vi "Periodic Tasks.vi"(8 "error in":errorcluster) -> ()   [LabVIEW 2019]
doc: "This VI runs in parallel to other tasks. It can contain as many user-defined periodic loops as you need. These can carry out PID or other sorts of timed response."
uses:
  <vilib>/Rock Robotics/WPI/ThirdParty/Phoenix-LabVIEW/Motor Controller/Controls/CTRE_Phoenix_MotorControl_ControlMode.ctl
  <vilib>/Rock Robotics/WPI/Utilities/WPI_GetSetVariantRefNum.vi
  <vilib>/Rock Robotics/Network Tables/NT Read Number.vi
  <vilib>/Rock Robotics/WPI/ThirdParty/Phoenix-LabVIEW/Motor Controller/Get/CTRE_Phoenix_MotorController_GetSupplyAndStatorCurrent_Enhanced.vi
  <vilib>/Rock Robotics/WPI/ThirdParty/Phoenix-LabVIEW/Motor Controller/Get/CTRE_Phoenix_MotorController_GetSelectedSensorData.vi
  <vilib>/gmath/NI_Gmath.lvlib
panel:
  in  "Output":dbl
  out "Target RPM":dbl
  out "Rpm":cluster{dbl, "Target RPM":dbl}(graph)
  out "Current":T1(graph)
  in  "PIDF Slot":i32
  in  "I-Zone":dbl
  in  "F":dbl=0.055
  in  "D":dbl
  in  "I":dbl
  in  "P":dbl
  out "Target Dist":dbl
  out "Outtake Sensor":bool
  out "Intake Sensor":bool
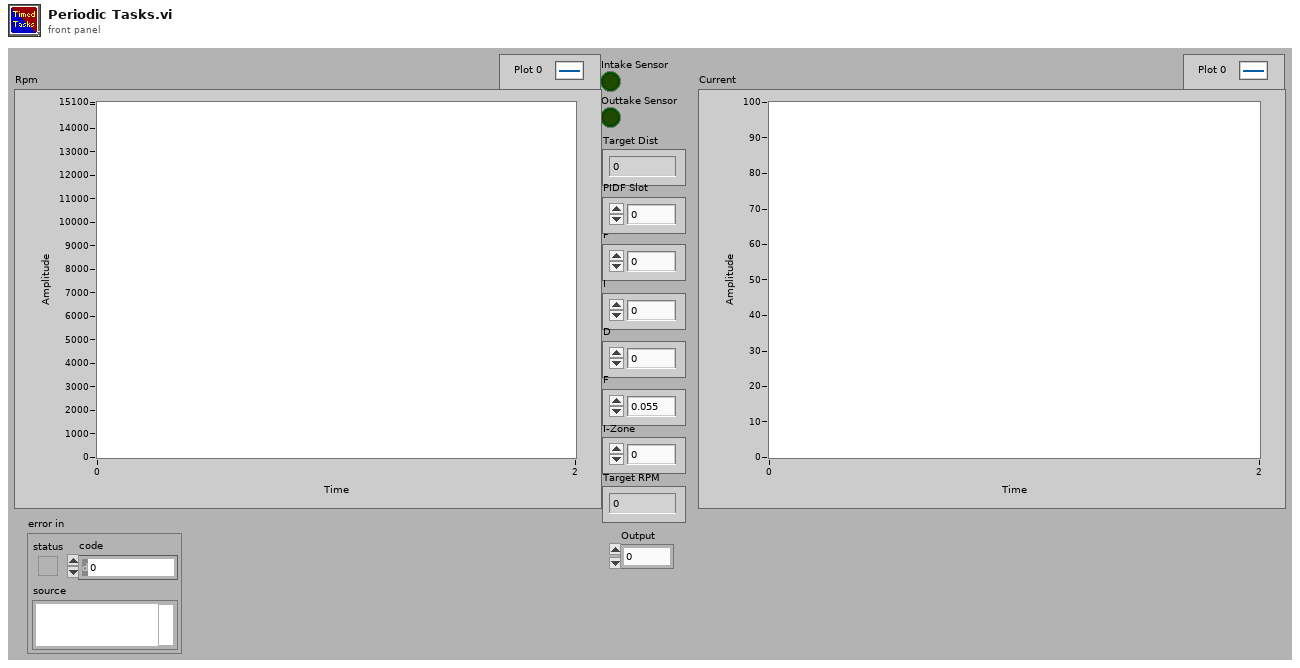
[diagram p1: front panel]
types:
  T1 = cluster{"Supply Current":dbl, "Stator Current":dbl}
  T2 = typedef "WPI_JoystickDevRef.ctl" = cluster{"Device":T3}
  T3 = typedef "WPI_JoystickDeviceEnum.ctl" = enum16{"USB 0", "USB 1", "USB 2", "USB 3", "USB 4", "USB 5"}
  T4 = typedef "WPI_MotorControlDeviceRef.ctl" = cluster{"DeviceStatus":errorcluster, "Type":T5, "PWM":cluster{"PWM Channel":T6, "DeadBand":T7}, "CAN":cluster{"Device Number":u8, "SetOutput VI Ref":variant, "GetOutput VI Ref":variant, "Enable VI Ref":variant, "Disable VI Ref":variant, "Data":variant}, "Invert":bool, "DIO PWM":cluster{"PWM \"Enable\" Channel":T6, "DIOChannel":T8, "PWM Rate":dbl}}
  T5 = typedef "WPI_MotorControlType.ctl" = enum16{"PWM", "CAN", "DIO PWM"}
  T6 = typedef "FPGA_DIOPWMChannel.ctl" = enum8{"PWM 0", "PWM 1", "PWM 2", "PWM 3", "PWM 4", "PWM 5", "PWM 6", "PWM 7", "PWM 8", "PWM 9", "PWM MXP 0", "PWM MXP 1", "PWM MXP 2", "PWM MXP 3", "PWM MXP 4", "PWM MXP 5", "PWM MXP 6", "PWM MXP 7", "PWM MXP 8", "PWM MXP 9", "Invalid"}
  T7 = typedef "WPI_PWMDeadband.ctl" = cluster{"Name":string, "maxPositivePwm":i32, "minPositivePwm":i32, "centerPwm":i32, "maxNegativePwm":i32, "minNegativePwm":i32, "angularRange":u16}
  T8 = typedef "FPGA_DIOChannel.ctl" = enum8{"DIO 0", "DIO 1", "DIO 2", "DIO 3", "DIO 4", "DIO 5", "DIO 6", "DIO 7", "DIO 8", "DIO 9", "DIO MXP 0", "DIO MXP 1", "DIO MXP 2", "DIO MXP 3", "DIO MXP 4", "DIO MXP 5", "DIO MXP 6", "DIO MXP 7", "DIO MXP 8", "DIO MXP 9", "DIO MXP 10", "DIO MXP 11", "DIO MXP 12", "DIO MXP 13", "DIO MXP 14", "DIO MXP 15", "SPI Port CS1", "SPI Port CS2", "SPI Port CS3", "SPI Port MISO", "SPI Port MOSI", "Invalid"}
  T9 = cluster{"PhoenixMotorControlDevRef":T4, "JoystickDevRef":T2}
  T10 = typedef "CTRE_Phoenix_MotorControl_ControlMode.ctl" = u16
  T11 = typedef "WPI_DigitalInputDevRef.ctl" = cluster{"DevStatus":errorcluster, "DIO Channel":T8}
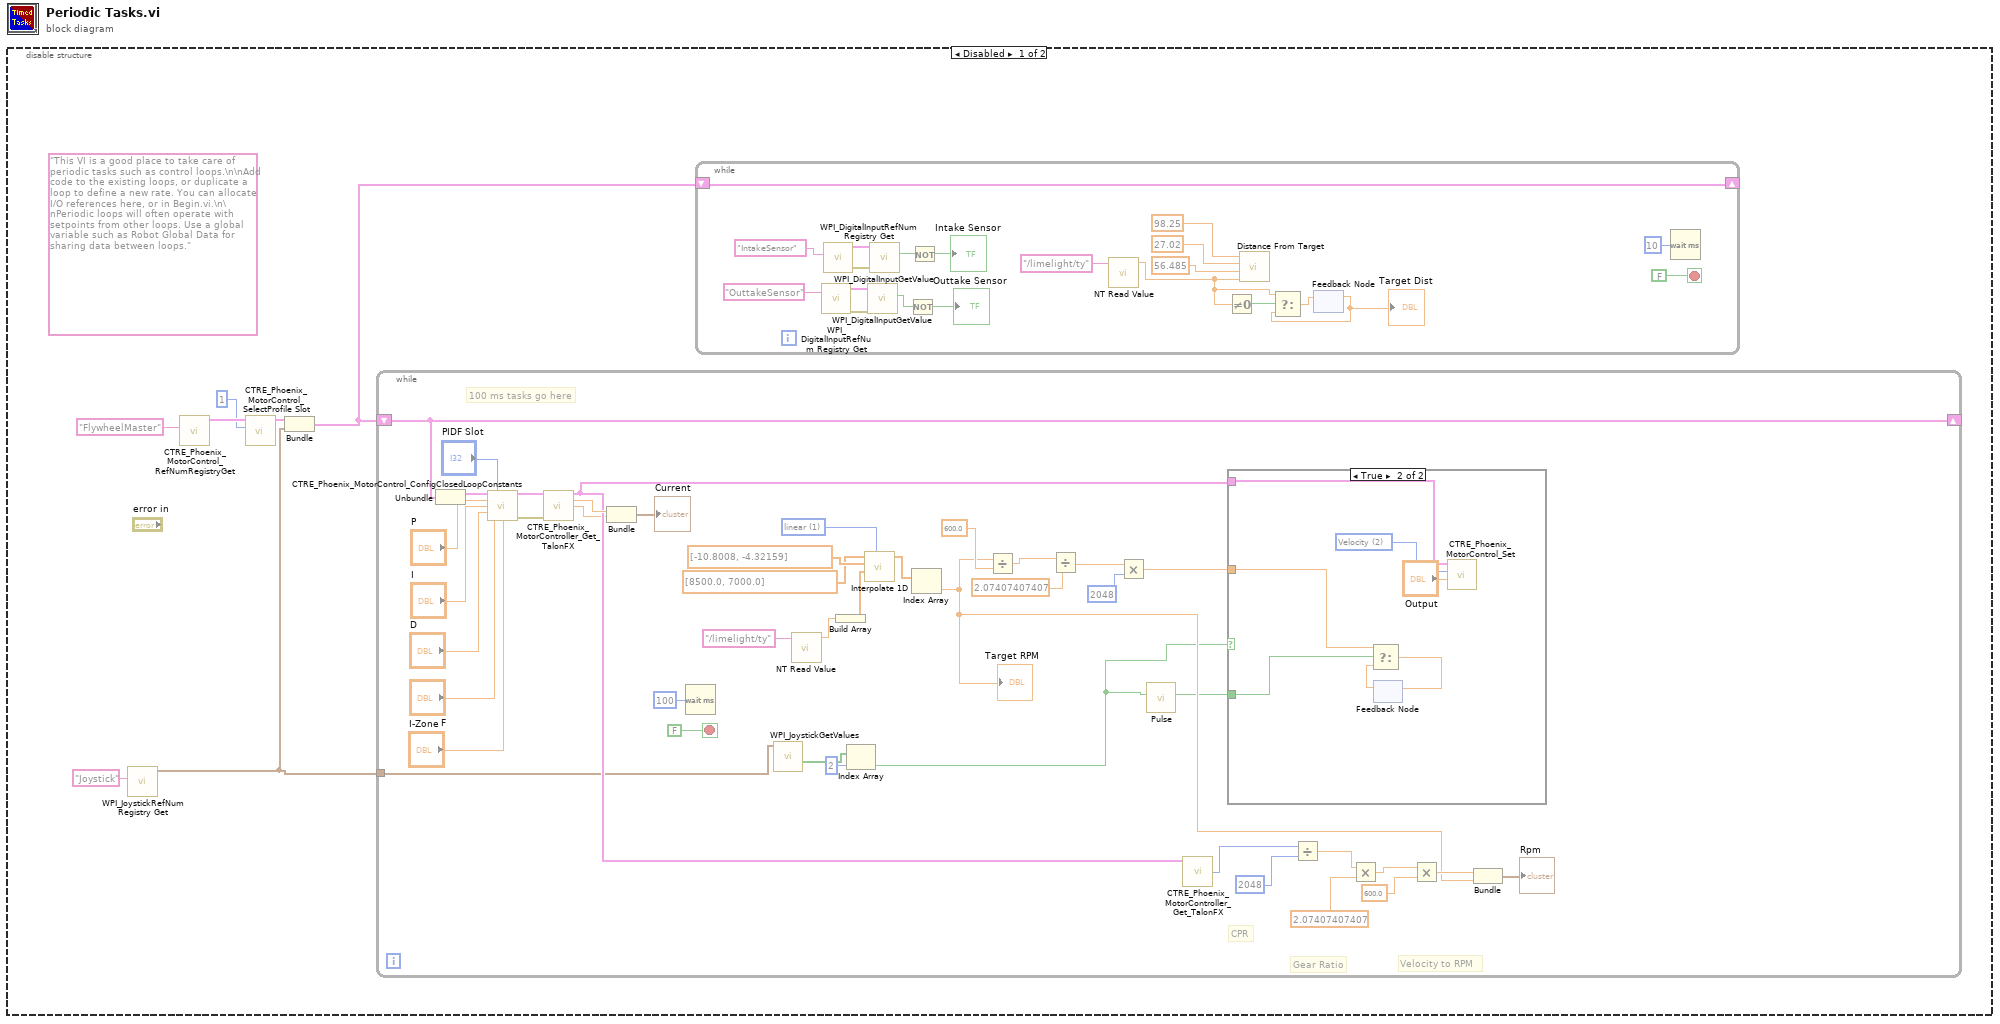
[diagram p0: block diagram]
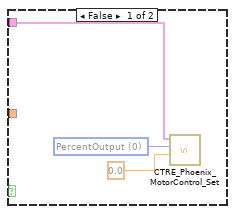
[diagram p2: hidden frame]
diagram:
  n1 = disable-structure shown="Disabled" {
    frame Disabled {
      (unwired) "This VI is a good place to take care of periodic tasks such as control loops.\n\nAdd code to the existing loops, or duplicate a loop to define a new rate. You can allocate I/O references here, or in Begin.vi.\n\nPeriodic loops will often operate with setpoints from other loops. Use a global variable such as Robot Global Data for sharing data between loops."
      n2 = call <vilib>:"WPI_JoystickRefNum Registry Get.vi"("refnum name"="Joystick") -> ("JoystickDevRef"=w1:T2)  [unwired: 9 in, 1 out]
      n3 = call <vilib>:"CTRE_Phoenix_MotorControl_RefNumRegistryGet.vi"("refnum name"="FlywheelMaster") -> ("PhoenixMotorControlDevRef"=w5:T4)  [unwired: 9 in, 1 out]
      n4 = call <vilib>:"CTRE_Phoenix_MotorControl_SelectProfile Slot.vi"("slotIdx"=1, "PhoenixMotorControlDevRef"=w5) -> ("PhoenixMotorControlDevRef"=w4:T4)  [unwired: 8 in, 1 out]
      n5 = Bundle("PhoenixMotorControlDevRef"=w4, "JoystickDevRef"=w1) -> (w7:T9)  [unwired: 1 out]
      n6 = while {
        shift-right: [w48] -> _
        shift-left: w7 -> [w48]
        tunnel: w1 -> [w13]
        stop <- FALSE stop-if-true
        w21 = 1 items=["nearest", "linear", "spline", "cubic Hermite", "Lagrange"] ("method")
        # "CPR"
        # "Velocity to RPM"
        # "Gear Ratio"
        # "100 ms tasks go here"
        n7 = Unbundle(w48) -> ("PhoenixMotorControlDevRef"=w47:T4)  [unwired: 1 out]
        n8 = call <vilib>:"CTRE_Phoenix_MotorControl_ConfigClosedLoopConstants.vi"("PhoenixMotorControlDevRef"=w47, "slotIdx"="PIDF Slot", "P"="P", "I"="I", "D"="D", "F"="F", "I Zone"="I-Zone") -> ("PhoenixMotorControlDevRef"=w40:T4, "error out"=w39:errorcluster)  [unwired: 7 in]
        n9 = call-poly <vilib>:"CTRE_Phoenix_MotorController_Get_TalonFX.vi"("PhoenixMotorControlDevRef"=w40, "error in"=w39) -> ("PhoenixMotorControlDevRef"=w36:T4, "Supply Current"=w37:dbl, "Stator Current"=w35:dbl)  [unwired: 10 in, 1 out]
        n10 = Bundle("Supply Current"=w37, "Stator Current"=w35) -> (→"Current":T1)  [unwired: 1 out]
        n11 = Wait (ms)(milliseconds to wait=u32 100) -> ()  [unwired: 1 out]
        n12 = call <vilib>:"WPI_JoystickGetValues.vi"("JoystickDevRef"=w13) -> ("Buttons"=w12:bool[])  [unwired: 6 in, 4 out]
        n13 = call-poly <vilib>:"NT Read Value.vi"("Name"="/limelight/ty") -> ("Numeric"=w19:dbl)  [unwired: 9 in, 1 out]
        n14 = Build Array(w19) -> (w18:dbl[])
        n15 = Index Array(array=w12, index=2) -> (element=w8:bool)
        n16 = call <vilib>:"Interpolate 1D.vi"("method"=w21, "xi"=w18, "X"=dbl[] [-10.8008, -4.32159], "Y"=dbl[] [8500.0, 7000.0]) -> ("yi"=w17:dbl[])  [unwired: 5 in, 2 out]
        n17 = Index Array(array=w17) -> (element=w14:dbl)  [unwired: 1 in]
        "Target RPM" <- w14
        n18 = Divide(x=w14, y=600.0) -> (x/y=w25:dbl)
        n19 = Divide(x=w25, y=2.07407407407) -> (x/y=w26:dbl)
        n20 = Multiply(x=w26, y=2048) -> (x*y=w10:dbl)
        n21 = call "Pulse.vi"("Input"=w8) -> ("Output"=w9:bool)  [unwired: 10 in]
        n22 = call-poly <vilib>:"CTRE_Phoenix_MotorController_Get_TalonFX.vi"("PhoenixMotorControlDevRef"=w36) -> ("Velocity (Raw Sensor Units per 100 ms)"=w31:i32)  [unwired: 11 in, 3 out]
        n23 = case shown="True" w8 {
          tunnel: w36 -> [w51 w59]
          tunnel: w10 -> [_ w58]
          tunnel: w9 -> [_ w55]
          frame False {
            w52 = T10 0 items=["PercentOutput"=0, "Position"=1, "Velocity"=2, "Current"=3, "Follower"=5, "MotionProfile"=6, "MotionMagic"=7, "MotionProfileArc"=10, "Disabled"=15] ("Control Mode")
            n24 = call <vilib>:"CTRE_Phoenix_MotorControl_Set.vi"("Output"=0.0, "Control Mode"=w52, "PhoenixMotorControlDevRef"=w51) -> ()  [unwired: 7 in, 2 out]
          }
          frame True {
            w60 = T10 2 items=["PercentOutput"=0, "Position"=1, "Velocity"=2, "Current"=3, "Follower"=5, "MotionProfile"=6, "MotionMagic"=7, "MotionProfileArc"=10, "Disabled"=15] ("Control Mode")
            n25 = feedback #1() -> (w57:dbl)  [unwired: 1 in]
            n26 = Select(t=w58, s=w55, f=w57) -> (s? t:f=w56:dbl)
            n27 = feedback-in #1(w56) -> ()
            n28 = call <vilib>:"CTRE_Phoenix_MotorControl_Set.vi"("Output"="Output", "Control Mode"=w60, "PhoenixMotorControlDevRef"=w59) -> ()  [unwired: 7 in, 2 out]
          }
        }
        n29 = Divide(x=w31, y=2048) -> (x/y=w30:dbl)
        n30 = Multiply(x=w30, y=2.07407407407) -> (x*y=w32:dbl)
        n31 = Multiply(x=w32, y=600.0) -> (x*y=w33:dbl)
        n32 = Bundle(w33, "Numeric"=w14) -> (→"Rpm":cluster{dbl, "Numeric":dbl})  [unwired: 1 out]
      }
      n33 = while {
        shift-right: [w65] -> _
        shift-left: w7 -> [w65]
        stop <- FALSE stop-if-true
        n34 = call <vilib>:"WPI_DigitalInputRefNum Registry Get.vi"("refnum name"="OuttakeSensor") -> ("error out"=w76:errorcluster, "DigitalInputDevRef"=w77:T11)  [unwired: 9 in]
        n35 = call <vilib>:"WPI_DigitalInputRefNum Registry Get.vi"("refnum name"="IntakeSensor") -> ("error out"=w79:errorcluster, "DigitalInputDevRef"=w78:T11)  [unwired: 9 in]
        n36 = call <vilib>:"WPI_DigitalInputGetValue.vi"("error in (no error)"=w76, "DigitalInputDevRef"=w77) -> ("Value"=w74:bool)  [unwired: 7 in, 2 out]
        n37 = call <vilib>:"WPI_DigitalInputGetValue.vi"("error in (no error)"=w79, "DigitalInputDevRef"=w78) -> ("Value"=w75:bool)  [unwired: 7 in, 2 out]
        n38 = Not(x=w74) -> (.not. x?=→"Outtake Sensor":bool)
        n39 = Not(x=w75) -> (.not. x?=→"Intake Sensor":bool)
        n40 = call-poly <vilib>:"NT Read Value.vi"("Name"="/limelight/ty") -> ("Numeric"=w62:dbl)  [unwired: 9 in, 1 out]
        n41 = Not Equal To 0?(x=w62) -> (x != 0?=w64:bool)
        n42 = call "Distance From Target.vi"("Target Angle (Deg)"=w62, "Camera Angle (Deg)"=56.485 ("Camera Angle"), "Camera Height (in)"=27.02, "Target Height (in)"=98.25 ("Camera Height (in)")) -> ()  [unwired: 1 out]
        n43 = feedback #2() -> (w61:dbl)  [unwired: 1 in]
        "Target Dist" <- w61
        n44 = Select(t=w62, s=w64, f=w61) -> (s? t:f=w63:dbl)
        n45 = feedback-in #2(w63) -> ()
        n46 = Wait (ms)(milliseconds to wait=u32 10) -> ()  [unwired: 1 out]
      }
    }
    frame Enabled {
    }
  }
